vi "Format.vi"(8 "error in (no error)":errorcluster, 10 "log record":T1 {"timestamp" format="%<%x %.3X>T"}, 11 "formatter in":refnum<class "Formatter.lvclass">) -> (0 "error out":errorcluster, 2 "log line":string, 3 "formatter out":refnum<class "Formatter.lvclass">)   [LabVIEW 2018, in "Logging.lvlib" / "Formatter.lvclass"]
uses:
  Formatter.lvclass
  Log Record.ctl
  Logger/Internal Log Levels.ctl
  Logging.lvlib
panel:
  # "Connector Pane"
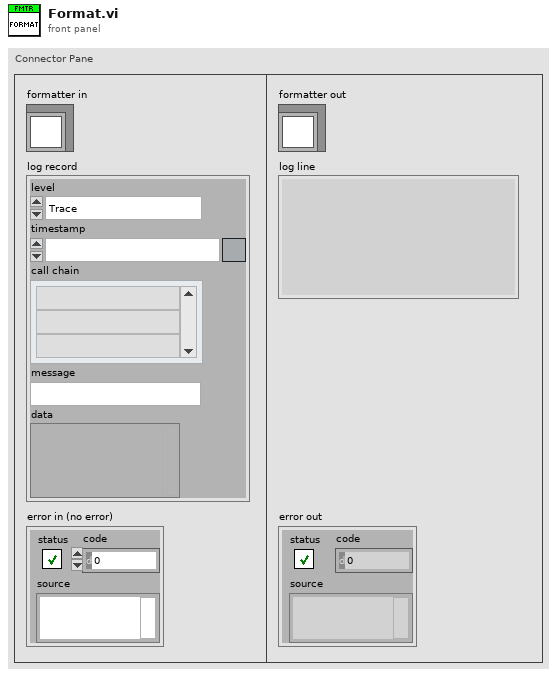
[diagram p1: front panel]
types:
  T1 = typedef "Logging.lvlib/Log Record.ctl" = cluster{"level":T2, "timestamp":timestamp, "call chain":string[], "message":string, "data":variant}
  T2 = typedef "Logging.lvlib/Internal Log Levels.ctl" = enum16{"Trace", "Debug", "Info", "Warning", "Error", "Critical", "Internal"}
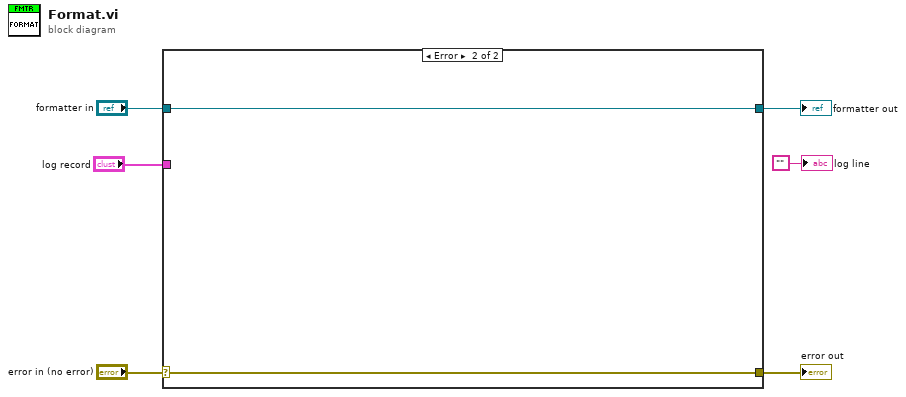
[diagram p0: block diagram]
diagram:
  n1 = case shown="Error" "error in (no error)" {
    selector: "error in (no error)" -> [w7 w10]
    tunnel: [w7 w10] -> w5
    tunnel: [w8 w9] -> w3
    tunnel: "formatter in" -> [w8 w9]
    tunnel: "log record" -> [_ _]
    frame No Error {
    }
    frame Error {
    }
  }
  "error out" <- w5
  "formatter out" <- w3
  "log line" <- ""
